vi "aquisicao_para_vibracao_do_acelerometro_triaxial.vi"() -> ()   [LabVIEW 2011]
uses:
  <vilib>/Waveform/WDTOps.llb/WDT Append Waveforms DBL.vi
panel:
  out "Vibração no eixo Z":dbl[](graph)
  out "Vibração no eixo Y":dbl[](graph)
  out "Vibração no eixo X":dbl[](graph)
  in  "Frequência de Amostragem":dbl
  in  "Botão \nGRAVAR":bool
  in  "Parar Programa":bool
  out "Sinal":waveform(dbl)[](graph) caption="DADOS"
  in  "Parar \naqusição":bool
  # "AQUISIÇÃO - PROPRIEDADES DINÂMICAS"
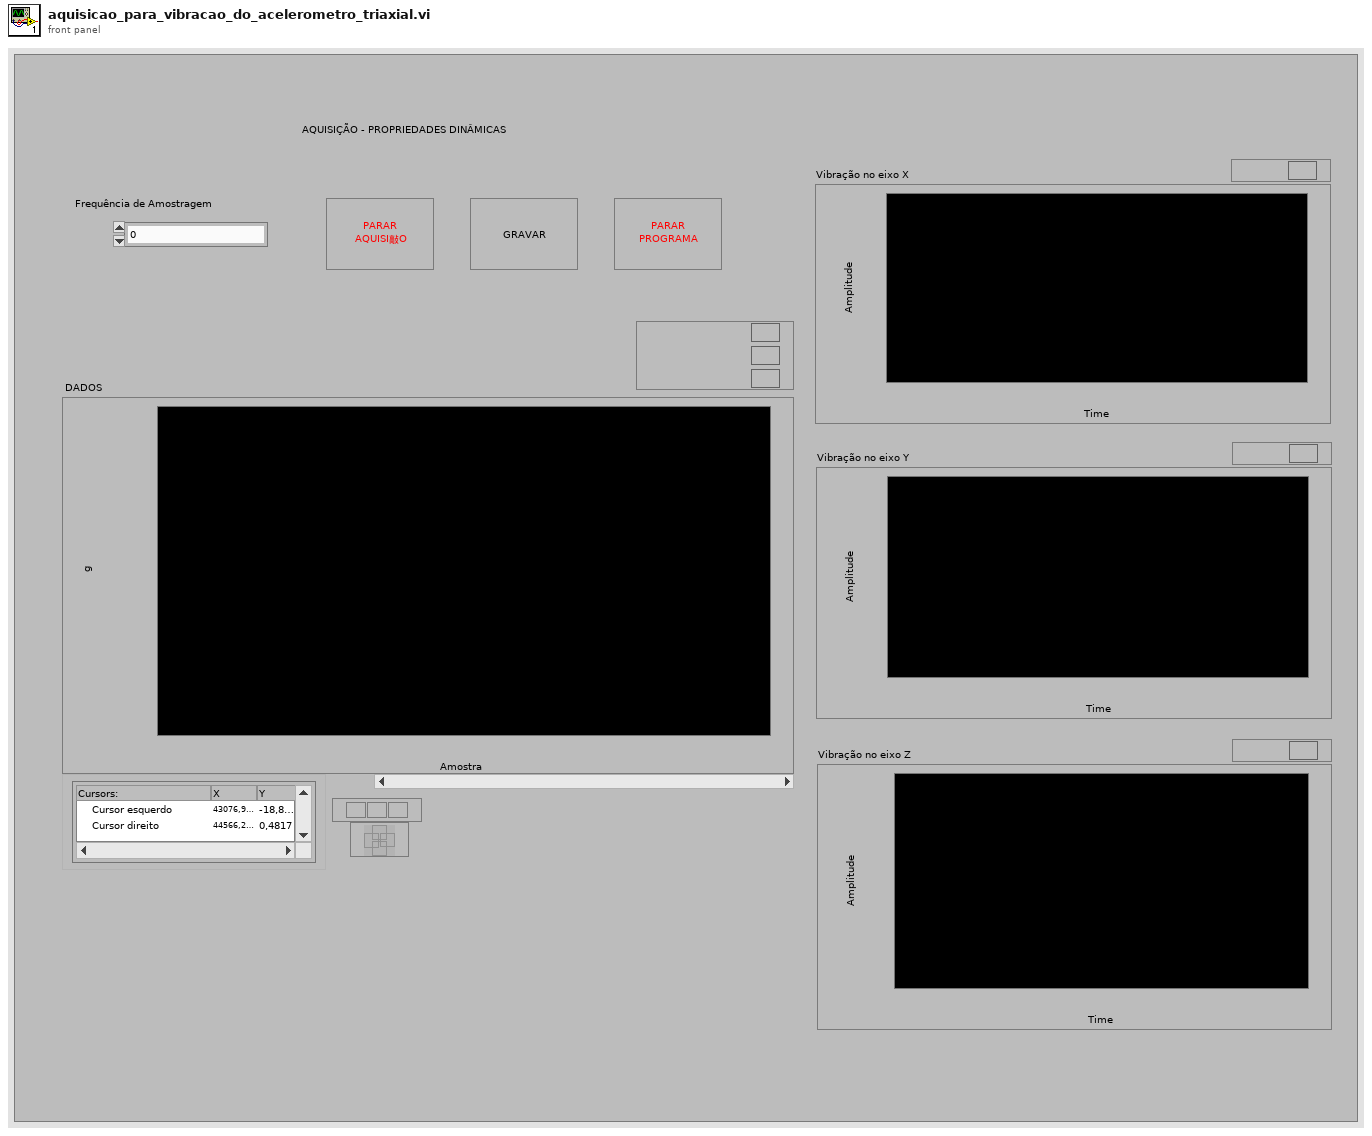
[diagram p1: front panel]
types:
  T1 = typedef "NI_Matrix.lvlib/RealMatrix.ctl" = dbl[][]
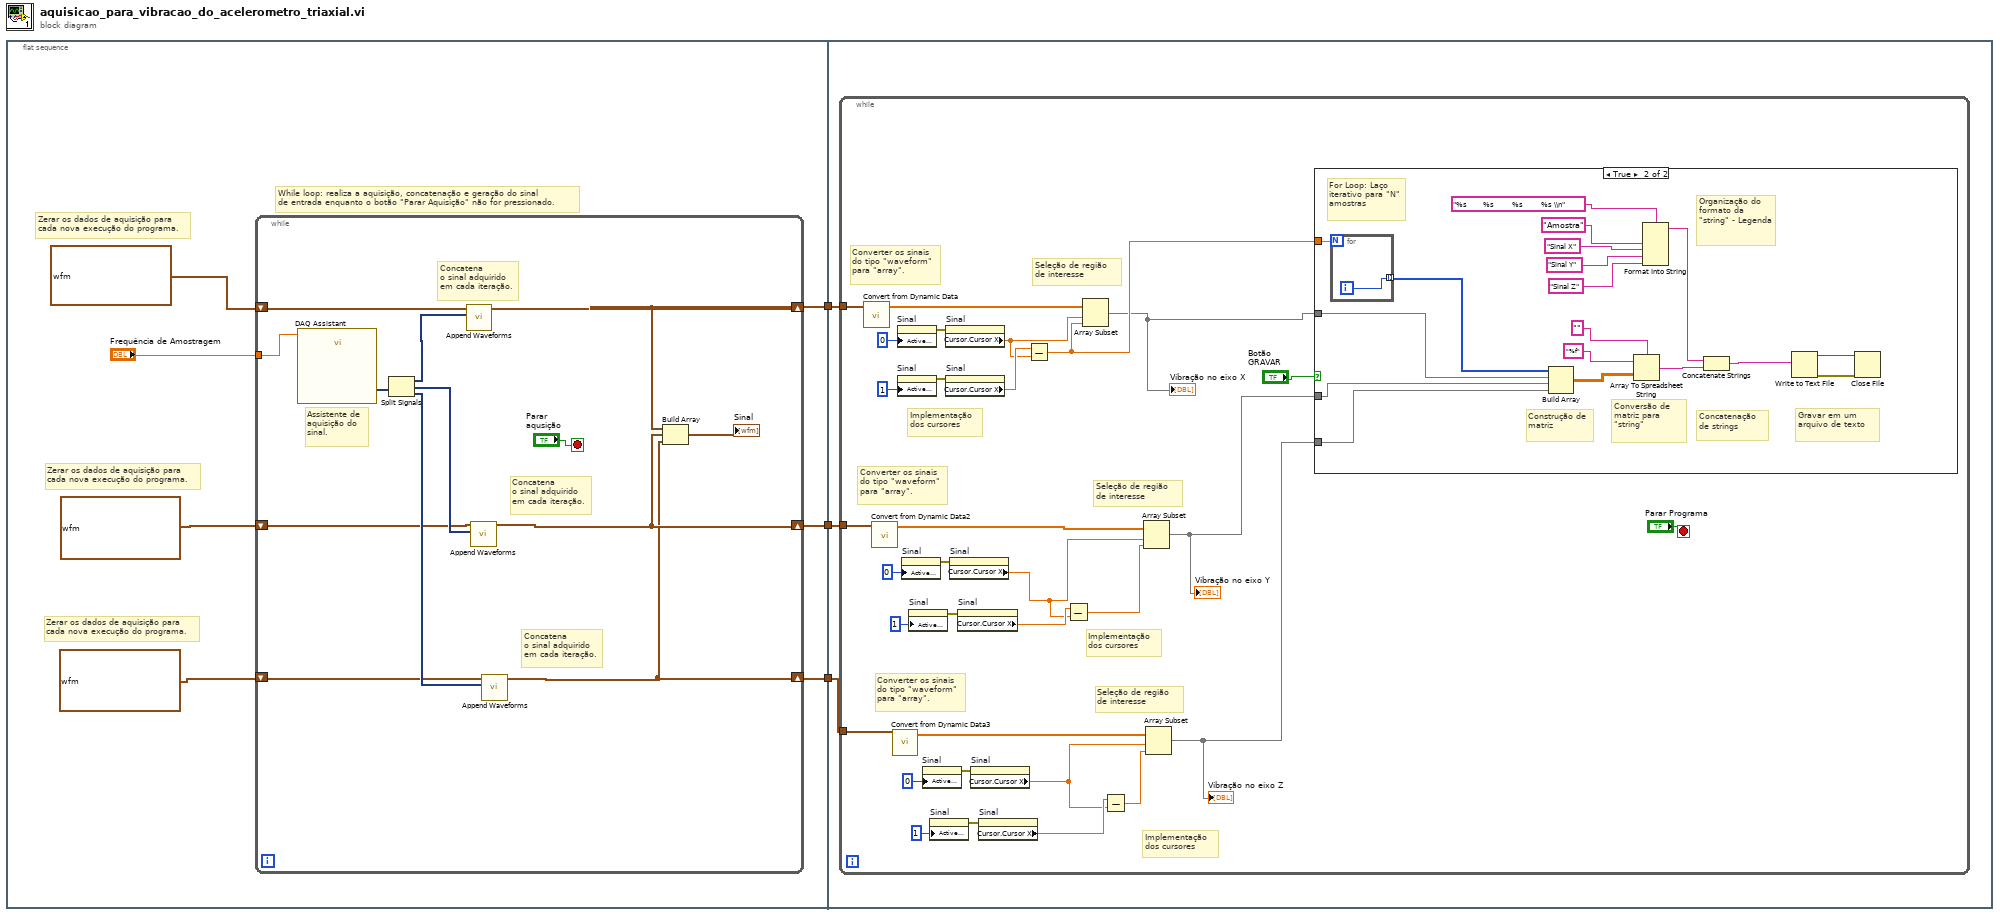
[diagram p0: block diagram]
diagram:
  n1 = flat-sequence {
    tunnel: [w9] -> w3
    tunnel: [w5] -> w2
    tunnel: [w4] -> w1
    tunnel: w3 -> [w26]
    tunnel: w2 -> [w25]
    tunnel: w1 -> [w24]
    frame #0 {
      # "Zerar os dados de aquisição para \ncada nova execução do programa."
      # "Zerar os dados de aquisição para \ncada nova execução do programa."
      # "Zerar os dados de aquisição para \ncada nova execução do programa."
      # "While loop: realiza a aquisição, concatenação e geração do sinal\nde entrada enquanto o botão \"Parar Aquisição\" não for pressionado."
      n2 = while "Aquisição do Sinal" {
        shift-right: [w13] -> w9
        shift-left: waveform(dbl) {"t0"=timestamp(0 s since 1904-01-01), "dt"=1.0, "Y"=[]} ("Waveform") -> [w22]
        tunnel: "Frequência de Amostragem" -> [w21]
        shift-right: [w12] -> w5
        shift-left: waveform(dbl) {"t0"=timestamp(0 s since 1904-01-01), "dt"=1.0, "Y"=[]} ("Waveform") -> [w16]
        shift-right: [w11] -> w4
        shift-left: waveform(dbl) {"t0"=timestamp(0 s since 1904-01-01), "dt"=1.0, "Y"=[]} ("Waveform") -> [w15]
        stop <- "Parar \naqusição" stop-if-true
        # "Concatena\no sinal adquirido\nem cada iteração."
        # "Concatena\no sinal adquirido\nem cada iteração."
        # "Assistente de \naquisição do\nsinal."
        # "Concatena\no sinal adquirido\nem cada iteração."
        n3 = call "DAQ Assistant"("rate"=w21) -> ("data"=w20:dynamicdata)  [unwired: 15 in, 3 out]
        n4 = Split Signals(w20) -> (w19:dynamicdata, w18:dynamicdata, w17:dynamicdata)  [unwired: 3 in]
        n5 = call-poly <vilib>:"Append Waveforms.vi"("waveform B"=w19, "waveform A"=w22) -> ("waveform out"=w13:waveform(dbl))  [unwired: 8 in, 1 out]
        n6 = call-poly <vilib>:"Append Waveforms.vi"("waveform B"=w18, "waveform A"=w16) -> ("waveform out"=w12:waveform(dbl))  [unwired: 8 in, 1 out]
        n7 = call-poly <vilib>:"Append Waveforms.vi"("waveform B"=w17, "waveform A"=w15) -> ("waveform out"=w11:waveform(dbl))  [unwired: 8 in, 1 out]
        n8 = Build Array(w13, w12, w11) -> (→"Sinal":waveform(dbl)[])
      }
    }
    frame #1 {
      n9 = while {
        tunnel: w26 -> [w52]
        tunnel: w25 -> [w46]
        tunnel: w24 -> [w44]
        stop <- "Parar Programa" stop-if-true
        # "Seleção de região de interesse"
        # "Implementação \ndos cursores"
        # "Converter os sinais\ndo tipo \"waveform\"\npara \"array\"."
        # "Seleção de região de interesse"
        # "Implementação \ndos cursores"
        # "Converter os sinais\ndo tipo \"waveform\"\npara \"array\"."
        # "Seleção de região de interesse"
        # "Implementação \ndos cursores"
        # "Converter os sinais\ndo tipo \"waveform\"\npara \"array\"."
        n10 = call "Convert from Dynamic Data"("Dynamic Data Type"=w52) -> ("Array"=w51:dbl[])  [unwired: 3 in]
        n11 = call "Convert from Dynamic Data2"("Dynamic Data Type"=w46) -> ("Array"=w47:dbl[])  [unwired: 3 in]
        n12 = call "Convert from Dynamic Data3"("Dynamic Data Type"=w44) -> ("Array"=w45:dbl[])  [unwired: 3 in]
        n13 = property on="Sinal" class="WFGraph (strict)"("Active Cursor"=u32 0) -> (error out=w58:errorcluster)  [unwired: 2 in, 1 out]
        n14 = property on="Sinal" class="WFGraph (strict)"("Active Cursor"=u32 1) -> (error out=w56:errorcluster)  [unwired: 2 in, 1 out]
        n15 = property on="Sinal" class="WFGraph (strict)"("Active Cursor"=u32 0) -> (error out=w43:errorcluster)  [unwired: 2 in, 1 out]
        n16 = property on="Sinal" class="WFGraph (strict)"("Active Cursor"=u32 1) -> (error out=w41:errorcluster)  [unwired: 2 in, 1 out]
        n17 = property on="Sinal" class="WFGraph (strict)"("Active Cursor"=u32 0) -> (error out=w39:errorcluster)  [unwired: 2 in, 1 out]
        n18 = property on="Sinal" class="WFGraph (strict)"("Active Cursor"=u32 1) -> (error out=w37:errorcluster)  [unwired: 2 in, 1 out]
        n19 = property on="Sinal" class="WFGraph (strict)"(error in=w58) -> ("Cursor.Cursor X"=w50:dbl)  [unwired: 1 in, 2 out]
        n20 = property on="Sinal" class="WFGraph (strict)"(error in=w56) -> ("Cursor.Cursor X"=w53:dbl)  [unwired: 1 in, 2 out]
        n21 = property on="Sinal" class="WFGraph (strict)"(error in=w43) -> ("Cursor.Cursor X"=w34:dbl)  [unwired: 1 in, 2 out]
        n22 = property on="Sinal" class="WFGraph (strict)"(error in=w41) -> ("Cursor.Cursor X"=w35:dbl)  [unwired: 1 in, 2 out]
        n23 = property on="Sinal" class="WFGraph (strict)"(error in=w39) -> ("Cursor.Cursor X"=w31:dbl)  [unwired: 1 in, 2 out]
        n24 = property on="Sinal" class="WFGraph (strict)"(error in=w37) -> ("Cursor.Cursor X"=w32:dbl)  [unwired: 1 in, 2 out]
        n25 = Subtract(x=w53, y=w50) -> (x-y=w48:dbl)
        n26 = Subtract(x=w35, y=w34) -> (x-y=w33:dbl)
        n27 = Array Subset(array=w51, index=w50, length=w48) -> (w29:dbl[])
        "Vibração no eixo X" <- w29
        n28 = Subtract(x=w32, y=w31) -> (x-y=w30:dbl)
        n29 = Array Subset(array=w47, index=w34, length=w33) -> (w28:dbl[])
        "Vibração no eixo Y" <- w28
        n30 = Array Subset(array=w45, index=w31, length=w30) -> (w27:dbl[])
        "Vibração no eixo Z" <- w27
        n31 = case shown="True" "Botão \nGRAVAR" {
          tunnel: w48 -> [_ w76]
          tunnel: w29 -> [_ w67]
          tunnel: w28 -> [_ w60]
          tunnel: w27 -> [_ w59]
          frame False {
          }
          frame True {
            # "Gravar em um arquivo de texto"
            # "Concatenação de strings"
            # "Organização do formato da \"string\" - Legenda"
            # "Conversão de matriz para \"string\""
            # "Construção de matriz"
            # "For Loop: Laço iterativo para \"N\" amostras"
            n32 = for {
              N: w76 -> [_]
              tunnel: [w77] -> w68 mode=indexing
              i -> [w77]
            }
            n33 = Build Array(w68, w67, w60, w59) -> (w66:T1)
            n34 = Array To Spreadsheet String(delimiter (Tab)="", array=w66, 3:"%f" ("format string")) -> (spreadsheet string=w70:string)
            n35 = Format Into String(format string="%s        %s         %s         %s \\n", "Amostra" ("input 1"), "Sinal X" ("input 2"), "Sinal Y" ("input 3"), "Sinal Z" ("input 4")) -> (resulting string=w69:string)  [unwired: 2 in, 1 out]
            n36 = Concatenate Strings(w69, w70) -> (w63:string)
            n37 = Write to Text File(text=w63) -> (refnum out=w65:refnum<file>, error out=w64:errorcluster)  [unwired: 3 in, 1 out]
            n38 = Close File(refnum=w65, error in=w64) -> ()  [unwired: 2 out]
          }
        }
      }
    }
  }
